vi "Read Created Attributes.vi"(10 "Alias":string, 11 "Base Actor in":refnum<class "Base Actor.lvclass">) -> (0 "Error out":errorcluster, 2 "Created Attributes":refnum<class "Attributes.lvclass">)   [LabVIEW 2020, in "jettl.lvlib" / "Actor.lvlib" / "Base Actor.lvclass"]
uses:
  Base Actor.lvclass
  Base Actor.lvclass/Base Actor.ctl
  Error/Error.lvlib
  Attributes/Attributes/Attributes.lvclass
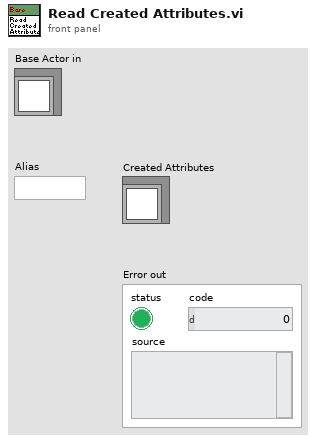
[diagram p1: front panel]
types:
  T1 = typedef "jettl.lvlib/Actor.lvlib/Base Actor.lvclass/Created Attributes Map.ctl" = map{string, refnum<class "Attributes.lvclass">}
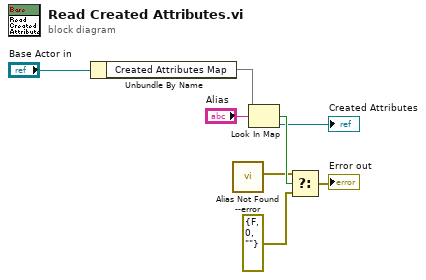
[diagram p0: block diagram]
diagram:
  n1 = Unbundle By Name("Base Actor in") -> ("Created Attributes Map"=w7:T1)
  n2 = call "Alias Not Found --error.vi"() -> ("Error"=w4:errorcluster)  [unwired: 11 in]
  n3 = Look In Map(map=w7, key="Alias") -> (key not found?=w5:bool, value=→"Created Attributes":refnum<class "Attributes.lvclass">)  [unwired: 1 in]
  n4 = Select(t=w4, s=w5, f=errorcluster {"status"=FALSE, "code"=0, "source"=""}) -> (s? t:f=→"Error out":errorcluster)
